vi "Volts to Binary Codes.vi"(0 "scaling coefficients":cluster{"gain":dbl, "offset":dbl}[](array[cluster]), 5 "channel index":u8, 7 "level (V)":dbl) -> (4 "codes":i16)   [LabVIEW 2015, in "Device Session.lvclass"]
doc: "Converts the voltage level for a channel source of a trigger block into ADC binary codes using the scaling coefficients for the particular channel source.\n\n<B>Input Parameters</B>\n\n<B>scaling coefficients</B> specifies the scaling coefficients used to convert the voltage level to codes for the particular channel source.\n\n<B>channel index</B> specifies the index of the channel used as the trigger source.\n\n<B>level (V)</B> specifies the trigger level to be converted.\n\n<B>Output Parameters</B>\n\n<B>codes</B> is the ADC code represented as a 16-bit integer. This value is converted from the voltage level using the gain and offset for the particular channel source."
uses:
  Device Session.lvclass
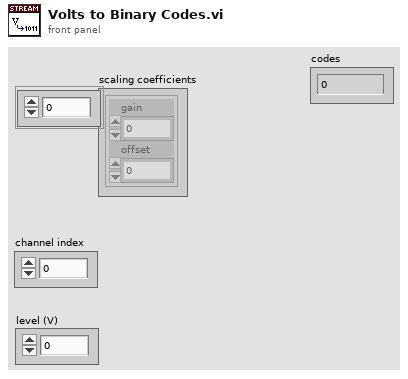
[diagram p1: front panel]
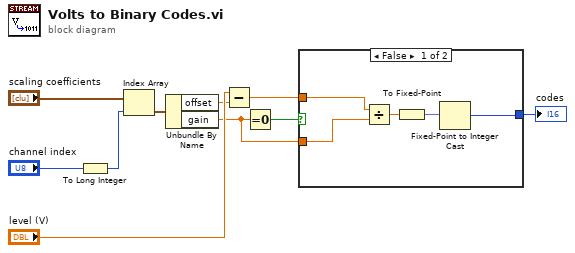
[diagram p0: block diagram]
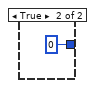
[diagram p2: hidden frame]
diagram:
  n1 = To Long Integer(number="channel index") -> (32bit integer=w2:i32)
  n2 = Index Array(array="scaling coefficients", index=w2) -> (element=w8:cluster{"gain":dbl, "offset":dbl})
  n3 = Unbundle By Name(w8) -> ("offset"=w7:dbl, "gain"=w4:dbl)
  n4 = Subtract(x="level (V)", y=w7) -> (x-y=w9:dbl)
  n5 = Equal To 0?(x=w4) -> (x = 0?=w6:bool)
  n6 = case shown="False" w6 {
    tunnel: w9 -> [w15 _]
    tunnel: [w11 i16 0] -> w5
    tunnel: w4 -> [w14 _]
    frame False {
      n7 = Divide(x=w15, y=w14) -> (x/y=w13:dbl)
      n8 = To Fixed-Point(number=w13) -> (fixed-point=w12:fxp<+/-,16,1>)  [unwired: 1 in]
      n9 = Fixed-Point to Integer Cast(1:w12) -> (0:w11:i16)
    }
    frame True {
    }
  }
  "codes" <- w5
